vi "SLM_Calibrator_MANUAL.vi"() -> ()   [LabVIEW 2011]
uses:
  <vilib>/userDefined/High Color/IMAQdx.ctl
  <vilib>/Utility/error.llb/DialogType.ctl
  <vilib>/vision/driver/NI_Vision_Acquisition_Software.lvlib
panel:
  in  "wait time (s)":u32=1
  in  "Tab Control":enum32{"CCD plane", "Plot"}(tab)
  out "Image Out":T1(plugin-control)
  out "XY Graph":cluster{dbl, dbl}[](graph)
  out "45º":bool
  out "135º":bool
  in  "Analizer":bool
  in  "Gradient2":bool
  in  "Gradient1":bool
  out "Yi2":dbl
  in  "Yc2":dbl(slide)=4.136690647482014 scale=0.0..10.0
  in  "Yf2:":dbl(slide)=5.467625899280575 scale=0.0..10.0
  out "Xi2":dbl
  in  "Xf2:":dbl(slide)=5.372670807453416 scale=0.0..10.0
  in  "Xc2":dbl(slide)=1.1180124223602483 scale=0.0..10.0
  out "CGH_y\nSLM2":T1(plugin-control)
  in  "Active1":bool=TRUE caption="Hide/Show (Show)"
  in  "Active2":bool=TRUE caption="Hide/Show (Show)"
  in  "STOP":bool caption="Stop (F)"
  out "PHASE":bool
  out "AMP":bool
  in  "amp_phase":bool
  out "SLM2 2":bool
  out "SLM1":bool
  in  "SLMs":bool=TRUE
  in  "Folter to save:":string
  out "Images done":dbl(slide) scale=0.0..256.0
  out "Yi1":dbl
  out "Xi1":dbl
  in  "Yf1:":dbl(slide)=5.5636363636363635 scale=0.0..10.0
  in  "Xf1:":dbl(slide)=6.5538461538461545 scale=0.0..10.0
  in  "Xc1":dbl(slide)=8.837920489296636 scale=0.0..10.0
  in  "Yc1":dbl(slide)=2.5818181818181816 scale=0.0..10.0
  out "CGH_x\nSLM1":T1(plugin-control)
  in  "Ready?\nCalibrate!":bool caption="Stop (F)"
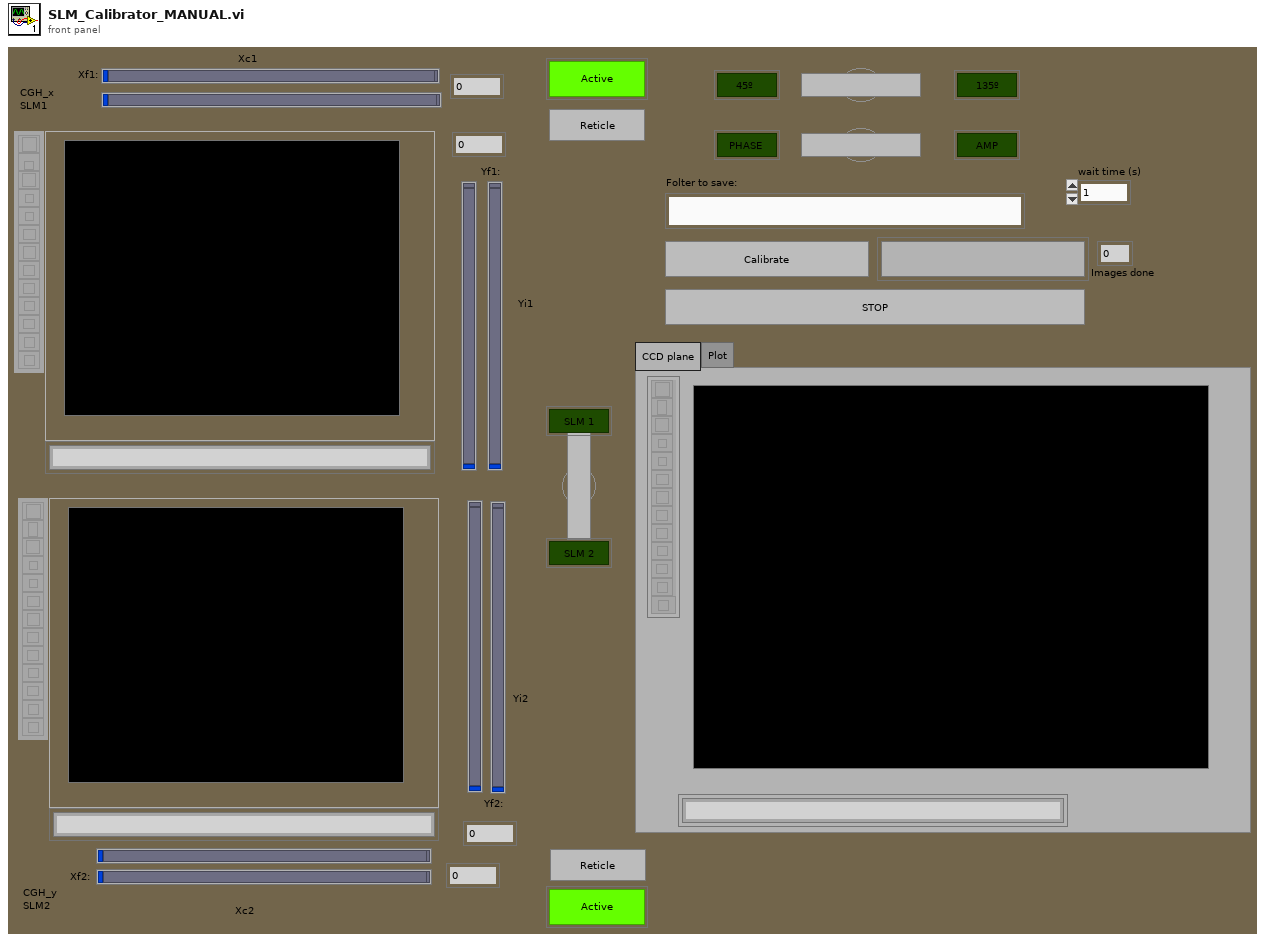
[diagram p1: front panel]
types:
  T1 = typedef "IMAQ Image.ctl" = refnum<image>
  T2 = typedef "IMAQdx.ctl" = refnum<k21>
  T3 = typedef "DialogType.ctl" = u16
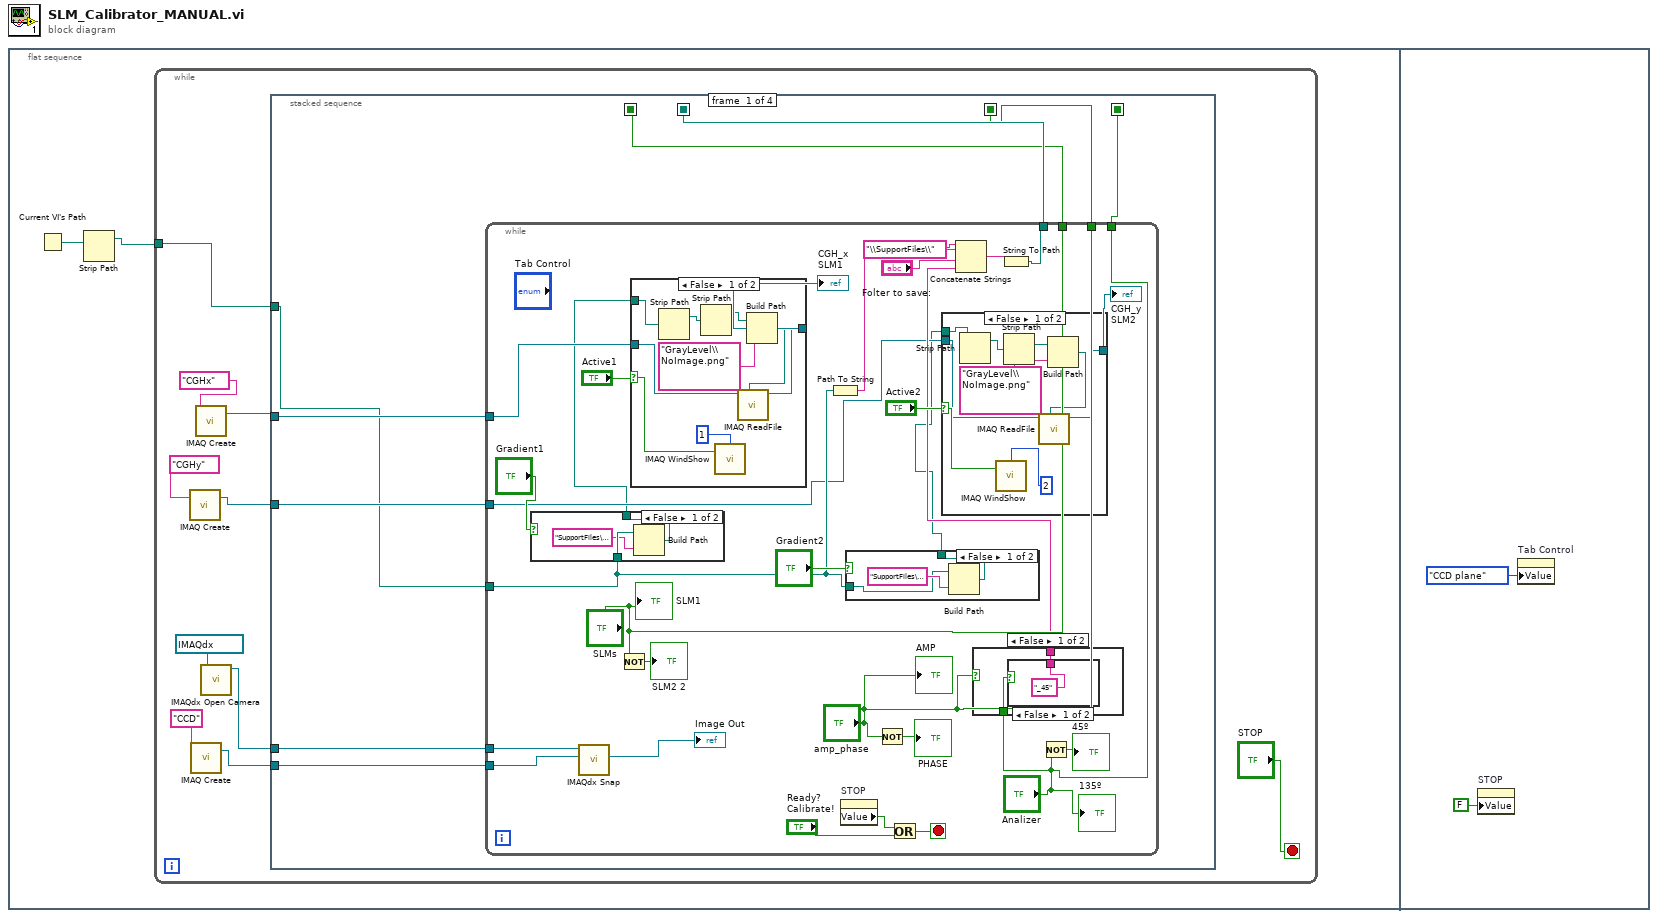
[diagram p0: block diagram]
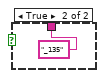
[diagram p2: hidden frame]
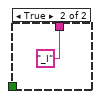
[diagram p3: hidden frame]
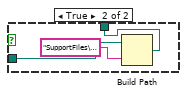
[diagram p4: hidden frame]
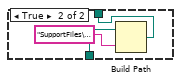
[diagram p5: hidden frame]
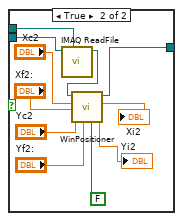
[diagram p6: hidden frame]
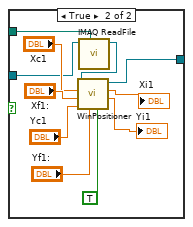
[diagram p7: hidden frame]
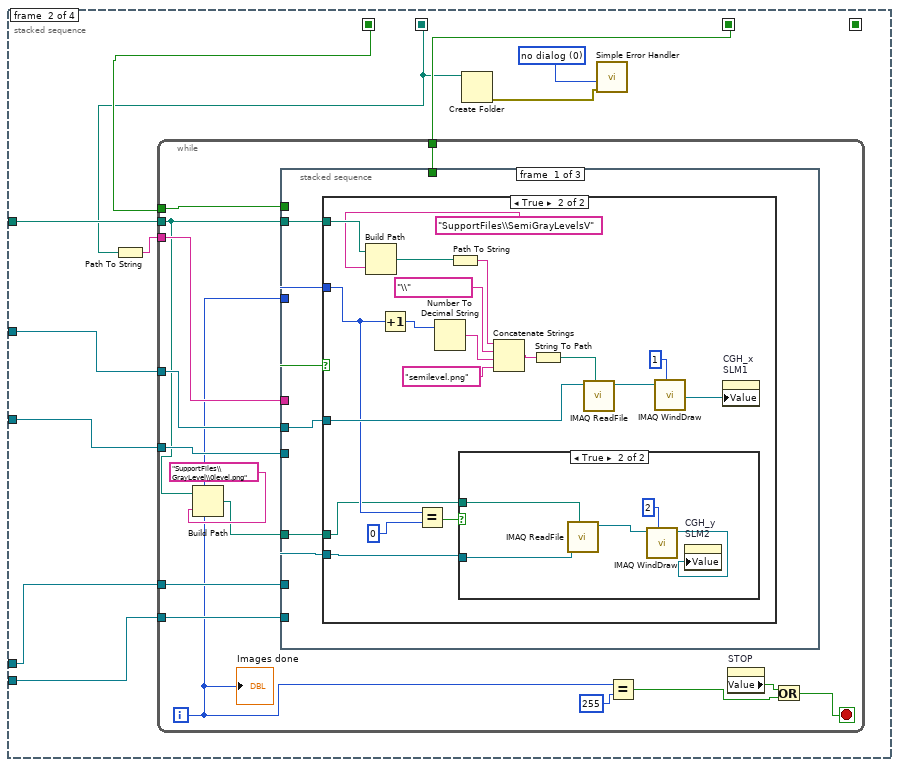
[diagram p8: hidden frame]
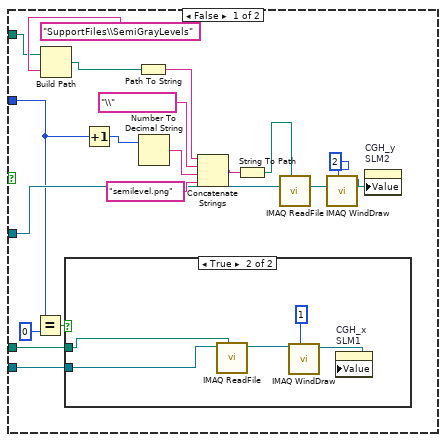
[diagram p9: hidden frame]
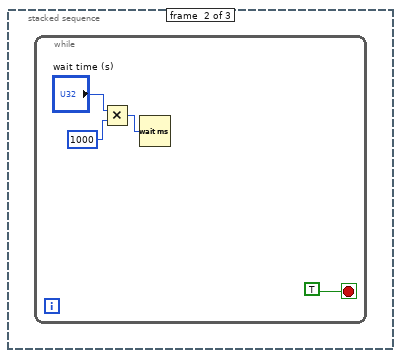
[diagram p12: hidden frame]
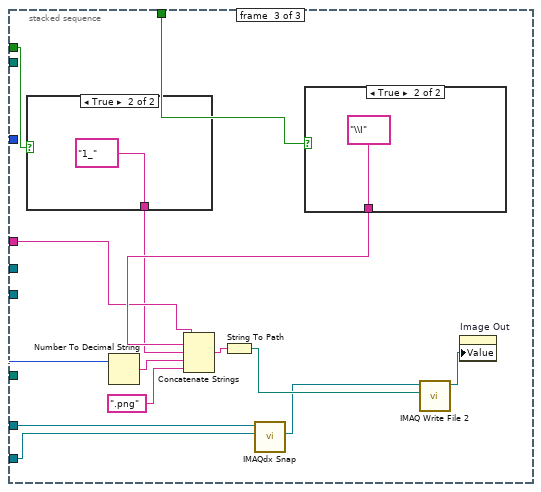
[diagram p13: hidden frame]
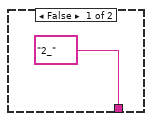
[diagram p14: hidden frame]
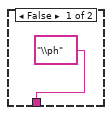
[diagram p15: hidden frame]
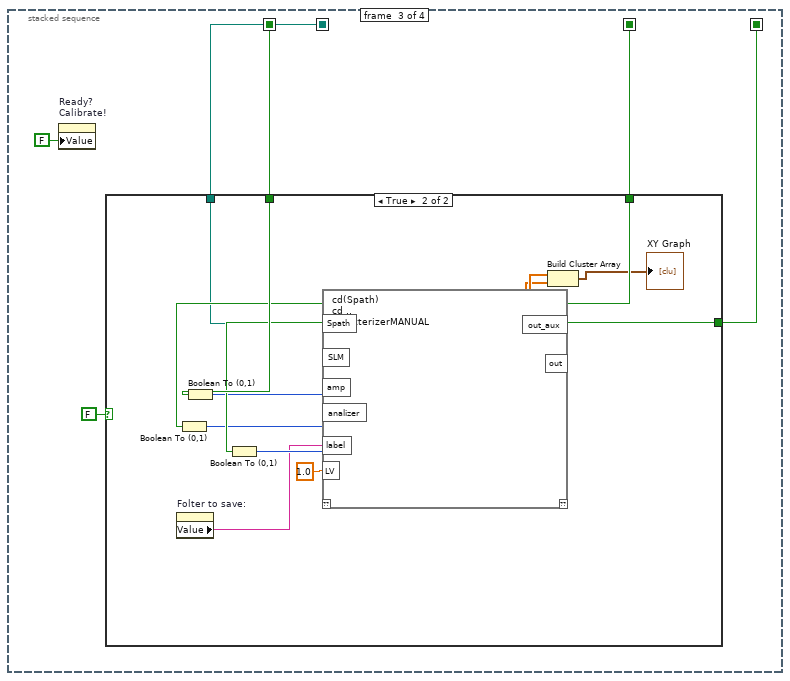
[diagram p16: hidden frame]
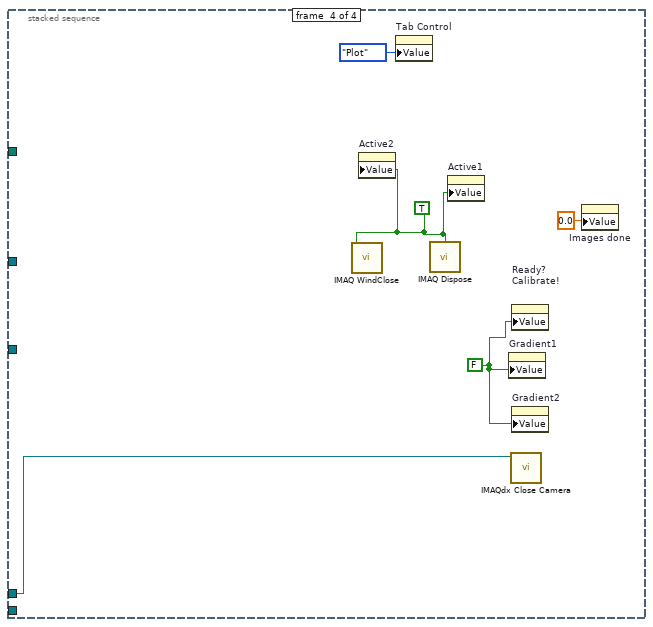
[diagram p18: hidden frame]
diagram:
  n1 = flat-sequence {
    frame #0 {
      n2 = Current VI's Path() -> (path=w2:path)
      n3 = Strip Path(path=w2) -> (stripped path=w1:path)  [unwired: 1 out]
      n4 = while {
        tunnel: w1 -> [w3]
        stop <- "STOP" stop-if-true
        n5 = call "IMAQ Create"("Image Name"="CGHy") -> ("New Image"=w7:T1)  [unwired: 4 in, 1 out]
        n6 = call "IMAQ Create"("Image Name"="CCD") -> ("New Image"=w6:T1)  [unwired: 4 in, 1 out]
        n7 = call "IMAQ Create"("Image Name"="CGHx") -> ("New Image"=w8:T1)  [unwired: 4 in, 1 out]
        n8 = call <vilib>:"IMAQdx Open Camera.vi"("Session In"=T2 "Paraxial") -> ("Session Out"=w5:T2)  [unwired: 9 in, 1 out]
        n9 = stacked-sequence {
          seq-local: [w19 _ _ _] -> [_ w110 w213 _]
          seq-local: [w17 _ _ _] -> [_ w114 w215 _]
          seq-local: [w18 _ _ _] -> [_ w115 w214 _]
          seq-local: [w13 _ _ _] -> [_ _ w212 _]
          tunnel: w7 -> [w15 w117 _ _]
          tunnel: w8 -> [w16 w118 _ _]
          tunnel: w5 -> [w21 w113 _ w229]
          tunnel: w6 -> [w20 w112 _ _]
          tunnel: w3 -> [w14 w111 _ _]
          frame #0 {
            n10 = while {
              tunnel: w21 -> [w48]
              tunnel: w20 -> [w47]
              tunnel: [w32] -> w19
              tunnel: ["amp_phase"] -> w18
              tunnel: ["SLMs"] -> w17
              tunnel: w16 -> [w23]
              tunnel: w15 -> [w25]
              tunnel: w14 -> [w31]
              tunnel: ["Analizer"] -> w13
              stop <- w44 stop-if-true
              n11 = case shown="False" "Gradient1" {
                tunnel: w31 -> [w64 w66]
                tunnel: [w62 w65] -> w22
                frame False {
                  n12 = Build Path(base path=w64, name or relative path="SupportFiles\\TestPatterns\\test_pattern.bmp") -> (appended path=w62:path)
                }
                frame True {
                  n13 = Build Path(base path=w66, name or relative path="SupportFiles\\TestPatterns\\test_pattern2V.png") -> (appended path=w65:path)
                }
              }
              n14 = call <vilib>:"IMAQdx Snap.vi"("Image In"=w47, "Session In"=w48) -> ("Image Out"=→"Image Out":T1)  [unwired: 7 in, 2 out]
              n15 = Not(x="SLMs") -> (.not. x?=→"SLM2 2":bool)
              n16 = case shown="False" "Active1" {
                selector: "Active1" -> [w96 _]
                tunnel: [w92 w100] -> w41
                tunnel: w23 -> [w90 w99]
                tunnel: w22 -> [w91 w97]
                frame False {
                  n17 = Strip Path(path=w91) -> (stripped path=w89:path)  [unwired: 1 out]
                  n18 = Strip Path(path=w89) -> (stripped path=w88:path)  [unwired: 1 out]
                  n19 = call "IMAQ WindShow"("Hide/Show (Show)"=w96, "Window Number (0...15)"=1) -> ()  [unwired: 4 in, 3 out]
                  n20 = Build Path(base path=w88, name or relative path="GrayLevel\\NoImage.png") -> (appended path=w93:path)
                  n21 = call "IMAQ ReadFile"("File Path"=w93, "Image"=w90) -> ("Image Out"=w92:T1)  [unwired: 5 in, 4 out]
                }
                frame True {
                  n22 = call "IMAQ ReadFile"("File Path"=w97, "Image"=w99) -> ("Image Out"=w98:T1)  [unwired: 5 in, 4 out]
                  n23 = call "WinPositioner.vi"("Image"=w98, "X position"="Xc1", "Fine X position"="Xf1:", "Y position"="Yc1", "Fine Y position"="Yf1:", "Display?"=TRUE) -> ("CGH_x"=w100:T1, "X position"=→"Xi1":dbl, "Y position"=→"Yi1":dbl)  [unwired: 2 in]
                }
              }
              "CGH_x\nSLM1" <- w41
              n24 = Path To String(path=w31) -> (string=w27:string)
              n25 = property on="STOP" class="Bool (strict)"() -> ("Value"=w43:bool)  [unwired: 2 in, 2 out]
              n26 = case shown="False" "Gradient2" {
                tunnel: [w57 w60] -> w24
                tunnel: w31 -> [w56 w59]
                frame False {
                  n27 = Build Path(base path=w56, name or relative path="SupportFiles\\TestPatterns\\test_pattern.bmp") -> (appended path=w57:path)
                }
                frame True {
                  n28 = Build Path(base path=w59, name or relative path="SupportFiles\\TestPatterns\\test_pattern2.png") -> (appended path=w60:path)
                }
              }
              n29 = Not(x="amp_phase") -> (.not. x?=→"PHASE":bool)
              n30 = Or(x=w43, y="Ready?\nCalibrate!") -> (x .or. y?=w44:bool)
              n31 = case shown="False" "Active2" {
                selector: "Active2" -> [w76 _]
                tunnel: [w70 w80] -> w39
                tunnel: w25 -> [w74 w78]
                tunnel: w24 -> [w73 w77]
                frame False {
                  n32 = Strip Path(path=w73) -> (stripped path=w69:path)  [unwired: 1 out]
                  n33 = call "IMAQ WindShow"("Hide/Show (Show)"=w76, "Window Number (0...15)"=2) -> ()  [unwired: 4 in, 3 out]
                  n34 = Strip Path(path=w69) -> (stripped path=w68:path)  [unwired: 1 out]
                  n35 = Build Path(base path=w68, name or relative path="GrayLevel\\NoImage.png") -> (appended path=w71:path)
                  n36 = call "IMAQ ReadFile"("File Path"=w71, "Image"=w74) -> ("Image Out"=w70:T1)  [unwired: 5 in, 4 out]
                }
                frame True {
                  n37 = call "IMAQ ReadFile"("File Path"=w77, "Image"=w78) -> ("Image Out"=w79:T1)  [unwired: 5 in, 4 out]
                  n38 = call "WinPositioner.vi"("Image"=w79, "X position"="Xc2", "Fine X position"="Xf2:", "Y position"="Yc2", "Fine Y position"="Yf2:", "Display?"=FALSE) -> ("CGH_x"=w80:T1, "X position"=→"Xi2":dbl, "Y position"=→"Yi2":dbl)  [unwired: 2 in]
                }
              }
              "CGH_y\nSLM2" <- w39
              n39 = case shown="False" "amp_phase" {
                tunnel: "Analizer" -> [w52 _]
                tunnel: [w51 "_I"] -> w28
                frame False {
                  n40 = case shown="False" w52 {
                    tunnel: ["_45" "_135"] -> w51
                    frame False {
                    }
                    frame True {
                    }
                  }
                }
                frame True {
                }
              }
              n41 = Concatenate Strings(w27, "\\SupportFiles\\" ("string"), "Folter to save:", w28) -> (w30:string)
              n42 = String To Path(string=w30) -> (path=w32:path)
              n43 = Not(x="Analizer") -> (.not. x?=→"45º":bool)
              "SLM1" <- "SLMs"
              "AMP" <- "amp_phase"
              "135º" <- "Analizer"
            }
          }
          frame #1 {
            w109 = T3 0 items=["no dialog", "OK message", "continue or stop message", "OK message + warnings", "continue/stop + warnings"] ("type of dialog (OK msg:1)")
            n44 = Path To String(path=w110) -> (string=w116:string)
            n45 = while {
              tunnel: w118 -> [w130]
              tunnel: w117 -> [w132]
              tunnel: w114 -> [w133]
              tunnel: w116 -> [w131]
              tunnel: w115 -> [w129]
              tunnel: w113 -> [w128]
              tunnel: w112 -> [w127]
              tunnel: w111 -> [w125]
              i -> [w121]
              stop <- w119 stop-if-true
              n46 = Build Path(base path=w125, name or relative path="SupportFiles\\GrayLevel\\0level.png") -> (appended path=w124:path)
              n47 = stacked-sequence {
                tunnel: w121 -> [w138 _ w201]
                tunnel: w131 -> [_ _ w200]
                tunnel: w133 -> [w139 _ w198]
                tunnel: w130 -> [w137 _ _]
                tunnel: w132 -> [w136 _ _]
                tunnel: w129 -> [_ _ w199]
                tunnel: w128 -> [_ _ w194]
                tunnel: w127 -> [_ _ w193]
                tunnel: w125 -> [w135 _ _]
                tunnel: w124 -> [w134 _ _]
                frame #0 {
                  n48 = case shown="True" w139 {
                    tunnel: w136 -> [w157 w173]
                    tunnel: w138 -> [w146 w169]
                    tunnel: w137 -> [w150 w172]
                    tunnel: w135 -> [w142 w167]
                    tunnel: w134 -> [w141 w164]
                    frame False {
                      n49 = Equal?(x=w146, y=0) -> (x = y?=w147:bool)
                      n50 = Build Path(base path=w142, name or relative path="SupportFiles\\SemiGrayLevels") -> (appended path=w144:path)
                      n51 = case shown="True" w147 {
                        tunnel: w157 -> [_ w162]
                        tunnel: w141 -> [_ w159]
                        frame False {
                        }
                        frame True {
                          n52 = call "IMAQ ReadFile"("File Path"=w159, "Image"=w162) -> ("Image Out"=w163:T1)  [unwired: 5 in, 4 out]
                          n53 = call "IMAQ WindDraw"("Window Number (0...15)"=1, "Image"=w163) -> ("Image Out (duplicate)"=w161:T1)  [unwired: 8 in, 1 out]
                          n54 = property on="CGH_x\nSLM1" class="ImageControl"("Value"=w161) -> ()  [unwired: 2 in, 2 out]
                        }
                      }
                      n55 = Increment(x=w146) -> (x+1=w153:i32)
                      n56 = Path To String(path=w144) -> (string=w155:string)
                      n57 = Number To Decimal String(number=w153) -> (decimal integer string=w154:string)  [unwired: 1 in]
                      n58 = Concatenate Strings(w155, "\\", w154, "semilevel.png") -> (w151:string)
                      n59 = String To Path(string=w151) -> (path=w149:path)
                      n60 = call "IMAQ ReadFile"("File Path"=w149, "Image"=w150) -> ("Image Out"=w158:T1)  [unwired: 5 in, 4 out]
                      n61 = call "IMAQ WindDraw"("Window Number (0...15)"=2, "Image"=w158) -> ("Image Out (duplicate)"=w140:T1)  [unwired: 8 in, 1 out]
                      n62 = property on="CGH_y\nSLM2" class="ImageControl"("Value"=w140) -> ()  [unwired: 2 in, 2 out]
                    }
                    frame True {
                      n63 = Build Path(base path=w167, name or relative path="SupportFiles\\SemiGrayLevelsV") -> (appended path=w165:path)
                      n64 = Increment(x=w169) -> (x+1=w176:i32)
                      n65 = Equal?(x=w169, y=0) -> (x = y?=w170:bool)
                      n66 = Number To Decimal String(number=w176) -> (decimal integer string=w177:string)  [unwired: 1 in]
                      n67 = Path To String(path=w165) -> (string=w178:string)
                      n68 = case shown="True" w170 {
                        tunnel: w173 -> [_ w185]
                        tunnel: w164 -> [_ w184]
                        frame False {
                        }
                        frame True {
                          n69 = call "IMAQ ReadFile"("File Path"=w184, "Image"=w185) -> ("Image Out"=w187:T1)  [unwired: 5 in, 4 out]
                          n70 = call "IMAQ WindDraw"("Window Number (0...15)"=2, "Image"=w187) -> ("Image Out (duplicate)"=w183:T1)  [unwired: 8 in, 1 out]
                          n71 = property on="CGH_y\nSLM2" class="ImageControl"("Value"=w183) -> ()  [unwired: 2 in, 2 out]
                        }
                      }
                      n72 = Concatenate Strings(w178, "\\", w177, "semilevel.png") -> (w174:string)
                      n73 = String To Path(string=w174) -> (path=w171:path)
                      n74 = call "IMAQ ReadFile"("File Path"=w171, "Image"=w172) -> ("Image Out"=w182:T1)  [unwired: 5 in, 4 out]
                      n75 = call "IMAQ WindDraw"("Window Number (0...15)"=1, "Image"=w182) -> ("Image Out (duplicate)"=w181:T1)  [unwired: 8 in, 1 out]
                      n76 = property on="CGH_x\nSLM1" class="ImageControl"("Value"=w181) -> ()  [unwired: 2 in, 2 out]
                    }
                  }
                }
                frame #1 {
                  n77 = while {
                    stop <- TRUE stop-if-true
                    n78 = Multiply(x="wait time (s)", y=u32 1000 ("milliseconds to wait 2")) -> (x*y=w188:u32)
                    n79 = Wait (ms)(milliseconds to wait=w188) -> ()  [unwired: 1 out]
                  }
                }
                frame #2 {
                  n80 = case shown="True" w198 {
                    tunnel: ["2_" "1_"] -> w197
                    frame False {
                    }
                    frame True {
                    }
                  }
                  n81 = Number To Decimal String(number=w201) -> (decimal integer string=w196:string)  [unwired: 1 in]
                  n82 = call <vilib>:"IMAQdx Snap.vi"("Image In"=w193, "Session In"=w194) -> ("Image Out"=w192:T1)  [unwired: 7 in, 2 out]
                  n83 = case shown="True" w199 {
                    tunnel: ["\\ph" "\\I"] -> w204
                    frame False {
                    }
                    frame True {
                    }
                  }
                  n84 = Concatenate Strings(w200, w204, w197, w196, ".png") -> (w203:string)
                  n85 = String To Path(string=w203) -> (path=w202:path)
                  n86 = call-poly "IMAQ Write File 2"("File Path"=w202, "Image"=w192) -> ("Image Out (duplicate)"=w205:T1)  [unwired: 8 in, 1 out]
                  n87 = property on="Image Out" class="ImageControl"("Value"=w205) -> ()  [unwired: 2 in, 2 out]
                }
              }
              n88 = Equal?(x=w121, y=255) -> (x = y?=w120:bool)
              n89 = property on="STOP" class="Bool (strict)"() -> ("Value"=w123:bool)  [unwired: 2 in, 2 out]
              n90 = Or(x=w123, y=w120) -> (x .or. y?=w119:bool)
              "Images done" <- w121
            }
            n91 = Create Folder(path (use dialog)=w110) -> (error out=w108:errorcluster)  [unwired: 2 in, 2 out]
            n92 = call <vilib>:"Simple Error Handler.vi"("type of dialog (OK msg:1)"=w109, "error in (no error)"=w108) -> ()  [unwired: 3 in, 5 out]
          }
          frame #2 {
            n93 = property on="Ready?\nCalibrate!" class="Bool (strict)"("Value"=FALSE ("Ready?\nCalibrate!")) -> ()  [unwired: 2 in, 2 out]
            n94 = case shown="True" FALSE {
              tunnel: w215 -> [_ w227]
              tunnel: w214 -> [_ w226]
              tunnel: w213 -> [_ w221]
              tunnel: w212 -> [_ w225]
              frame False {
              }
              frame True {
                n95 = property on="Folter to save:" class="Str"() -> ("Value"=w217:string)  [unwired: 2 in, 2 out]
                n96 = Boolean To (0,1)(Boolean=w226) -> (0, 1=w223:i16)
                n97 = Boolean To (0,1)(Boolean=w227) -> (0, 1=w224:i16)
                n98 = Boolean To (0,1)(Boolean=w225) -> (0, 1=w222:i16)
                n99 = script code="cd(Spath)\ncd ..\ncaracterizerMANUAL"("SLM"=w224, "amp"=w223, "Spath"=w221, "analizer"=w222, "label"=w217, "LV"=1.0 ("Real")) -> ("out"=w219:dbl[], "out_aux"=w220:dbl[])  [unwired: 1 in, 1 out]
                n100 = Build Cluster Array(w220, w219) -> (→"XY Graph":cluster{dbl, dbl}[])
              }
            }
          }
          frame #3 {
            w230 = TRUE ("Close All Windows (False)")
            w231 = FALSE ("Ready?\nCalibrate!")
            n101 = call "IMAQ WindClose"("Close All Windows (False)"=w230) -> ()  [unwired: 5 in, 1 out]
            n102 = property on="Active2" class="Bool (strict)"("Value"=w230) -> ()  [unwired: 2 in, 2 out]
            n103 = property on="Tab Control" class="TabCtl (strict)"("Value"=enum32{"CCD plane", "Plot"}."Plot" ("Tab Control")) -> ()  [unwired: 2 in, 2 out]
            n104 = call "IMAQ Dispose"("All Images? (No)"=w230) -> ()  [unwired: 5 in, 1 out]
            n105 = property on="Active1" class="Bool (strict)"("Value"=w230) -> ()  [unwired: 2 in, 2 out]
            n106 = property on="Gradient1" class="Bool (strict)"("Value"=w231) -> ()  [unwired: 2 in, 2 out]
            n107 = call <vilib>:"IMAQdx Close Camera.vi"("Session In"=w229) -> ()  [unwired: 10 in, 1 out]
            n108 = property on="Ready?\nCalibrate!" class="Bool (strict)"("Value"=w231) -> ()  [unwired: 2 in, 2 out]
            n109 = property on="Gradient2" class="Bool (strict)"("Value"=w231) -> ()  [unwired: 2 in, 2 out]
            n110 = property on="Images done" class="Slide (strict)"("Value"=0.0 ("Images done")) -> ()  [unwired: 2 in, 2 out]
          }
        }
      }
    }
    frame #1 {
      n111 = property on="STOP" class="Bool (strict)"("Value"=FALSE ("STOP")) -> ()  [unwired: 2 in, 2 out]
      n112 = property on="Tab Control" class="TabCtl (strict)"("Value"=enum32{"CCD plane", "Plot"}."CCD plane" ("Tab Control")) -> ()  [unwired: 2 in, 2 out]
    }
  }
